vi "LWXPS_MultipleAxesPVTPulseOutputSet.vi"(5 "LabVIEW error IN":errorcluster, 6 "XPS Reference IN":refnum<k24>, 7 "Time Interval":dbl, 8 "End Element":i32, 9 "Start Element":i32, 10 "Group Name":string) -> (0 "LabVIEW error OUT":errorcluster, 1 "XPS Error String":string, 2 "Returned error code":i32, 3 "XPS Reference OUT":refnum<k24>)   [LabVIEW 2014]
uses:
  D:/XPSQ8_LabView_Library/Development/Source/Dll/Newport.XPS.CommandInterface.dll
  Dll/Newport.XPS.CommandInterface.dll
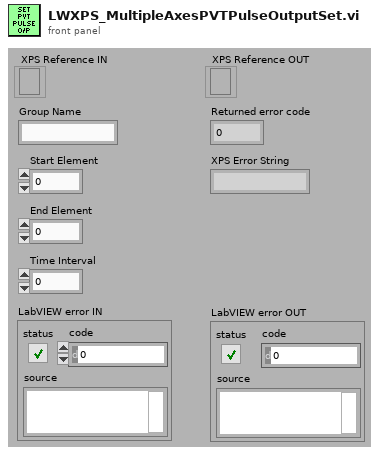
[diagram p1: front panel]
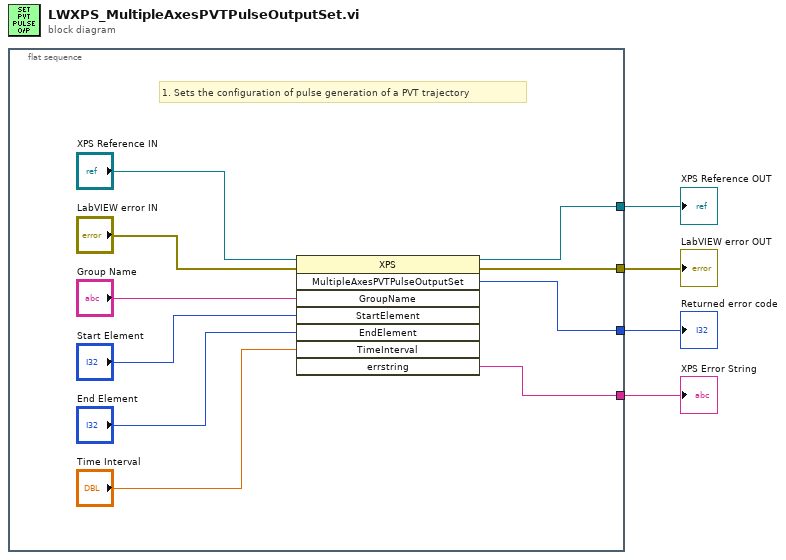
[diagram p0: block diagram]
diagram:
  n1 = flat-sequence {
    tunnel: [w12] -> w4
    tunnel: [w14] -> w3
    tunnel: [w11] -> w2
    tunnel: [w8] -> w1
    frame #0 {
      # "1. Sets the configuration of pulse generation of a PVT trajectory"
      n2 = invoke class="XPS" method="MultipleAxesPVTPulseOutputSet"(reference="XPS Reference IN", error in="LabVIEW error IN", "GroupName"="Group Name", "StartElement"="Start Element", "EndElement"="End Element", "TimeInterval"="Time Interval") -> (reference out=w12:refnum<k24>, error out=w14:errorcluster, "MultipleAxesPVTPulseOutputSet"=w11:i32, "errstring"=w8:string)  [unwired: 2 in, 4 out]
    }
  }
  "XPS Reference OUT" <- w4
  "LabVIEW error OUT" <- w3
  "Returned error code" <- w2
  "XPS Error String" <- w1
